vi "TeslaVelox_getCoordinateSystem.vi"(11 "TeslaVeloxProbeStation.lvclass":refnum<class "TeslaVeloxProbeStation.lvclass">) -> (3 "Coordinate system":enum16{"Cartesian", "X as index"}(ring))   [LabVIEW 2018, in "TeslaVeloxProbeStation.lvclass"]
uses:
  TeslaVeloxProbeStation.lvclass
  TeslaVeloxProbeStation.lvclass/TeslaVeloxProbeStation.ctl
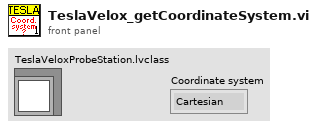
[diagram p1: front panel]
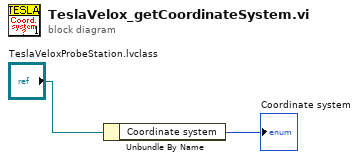
[diagram p0: block diagram]
diagram:
  n1 = Unbundle By Name("TeslaVeloxProbeStation.lvclass") -> ("Coordinate system"=→"Coordinate system":enum16{"Cartesian", "X as index"})
